vi "convert2cluster.vi"(6 "Measurement CH type":string, 7 "Input CH type":string, 8 "Sampling time":string, 9 "Final value":string, 10 "Initial value":string, 11 "Interval time":string) -> (3 "element":T1 {"Meas. CH Type" items=["Current", "Voltage", ""]; "Input CH Type" items=["Current", "Voltage", ""]})   [LabVIEW 2012]
uses:
  controls/MeasurementType.ctl
  controls/KeithlyChannelType.ctl
  controls/KeithlyFunction.ctl
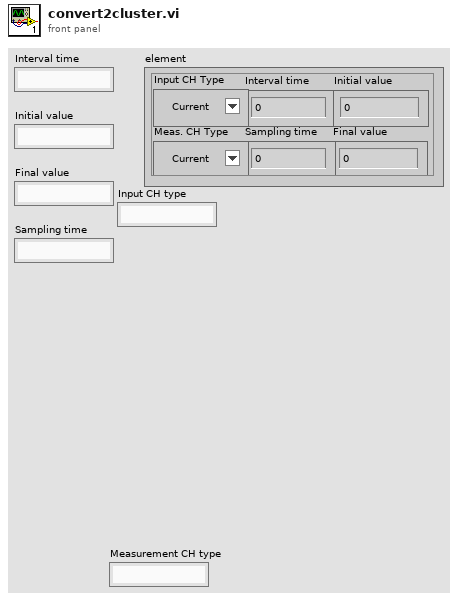
[diagram p1: front panel]
types:
  T1 = typedef "KeithlyFunction.ctl" = cluster{"Interval time":dbl, "Input CH Type":T2, "Initial value":dbl, "Final value":dbl, "Sampling time":dbl, "Meas. CH Type":T3}
  T2 = typedef "KeithlyChannelType.ctl" = u16
  T3 = typedef "MeasurementType.ctl" = u16
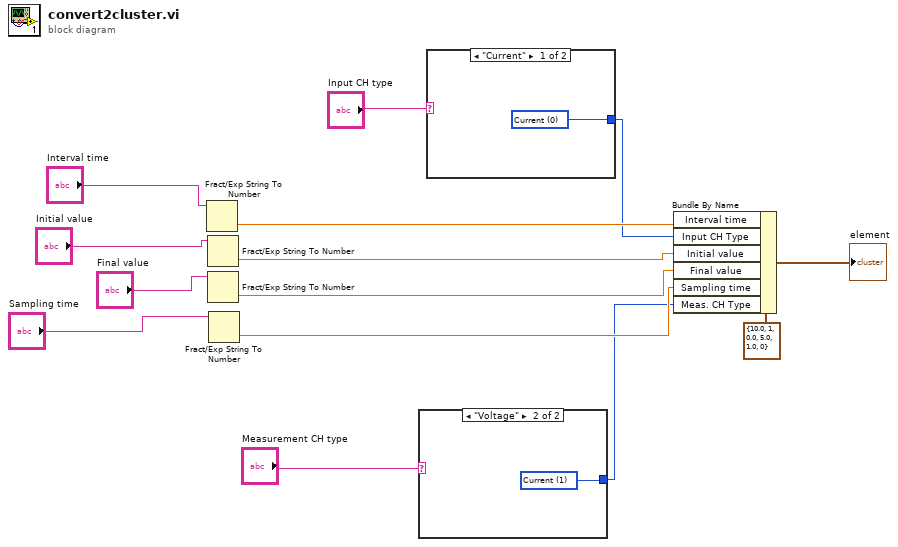
[diagram p0: block diagram]
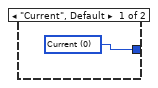
[diagram p2: hidden frame]
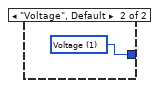
[diagram p3: hidden frame]
diagram:
  n1 = Fract/Exp String To Number(string="Interval time") -> (number=w6:dbl)  [unwired: 3 in, 1 out]
  n2 = Fract/Exp String To Number(string="Initial value") -> (number=w7:dbl)  [unwired: 3 in, 1 out]
  n3 = Fract/Exp String To Number(string="Final value") -> (number=w8:dbl)  [unwired: 3 in, 1 out]
  n4 = Fract/Exp String To Number(string="Sampling time") -> (number=w12:dbl)  [unwired: 3 in, 1 out]
  n5 = case shown="\"Voltage\"" "Measurement CH type" {
    tunnel: [w15 w16] -> w1
    frame "Current", Default {
      w15 = T3 0 items=["Current", "Voltage"] ("Meas. CH Type")
    }
    frame "Voltage" {
      w16 = T3 1 items=["Voltage", "Current"] ("Meas. CH Type")
    }
  }
  n6 = case shown="\"Current\"" "Input CH type" {
    tunnel: [w17 w18] -> w3
    frame "Current" {
      w17 = T2 0 items=["Current", "Voltage", ""] ("Input CH Type")
    }
    frame "Voltage", Default {
      w18 = T2 1 items=["Current", "Voltage", ""] ("Input CH Type")
    }
  }
  n7 = Bundle By Name(cluster=T1 {"Interval time"=10.0, "Input CH Type"=1, "Initial value"=0.0, "Final value"=5.0, "Sampling time"=1.0, "Meas. CH Type"=0} ("element"), "Interval time"=w6, "Input CH Type"=w3, "Initial value"=w7, "Final value"=w8, "Sampling time"=w12, "Meas. CH Type"=w1) -> (→"element":T1)
